vi "Write StreamChannels.vi"(8 "error in (no error)":errorcluster, 10 "StreamChannels":string[](array[string]), 11 "WaveformAcq configuration in":refnum<class "WaveformAcq configuration.lvclass">) -> (0 "error out":errorcluster, 3 "WaveformAcq configuration out":refnum<class "WaveformAcq configuration.lvclass">)   [LabVIEW 2017, in "WaveformAcq configuration.lvclass"]
uses:
  WaveformAcq configuration.lvclass
  WaveformAcq configuration.lvclass/WaveformAcq configuration.ctl
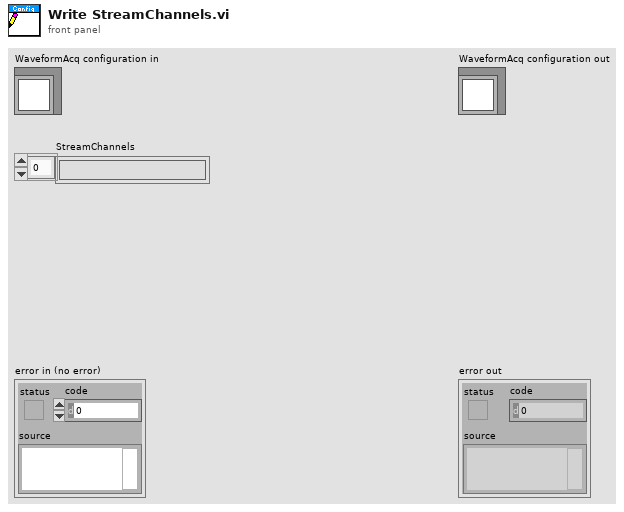
[diagram p1: front panel]
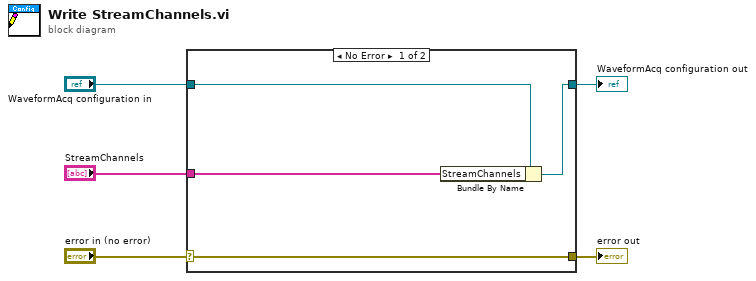
[diagram p0: block diagram]
diagram:
  n1 = case shown="No Error" "error in (no error)" {
    selector: "error in (no error)" -> [w9 w10]
    tunnel: [w9 w10] -> w4
    tunnel: [w7 w11] -> w2
    tunnel: "WaveformAcq configuration in" -> [w8 w11]
    tunnel: "StreamChannels" -> [w6 _]
    frame No Error {
      n2 = Bundle By Name(cluster=w8, "StreamChannels"=w6) -> (w7:refnum<class "WaveformAcq configuration.lvclass">)
    }
    frame Error {
    }
  }
  "error out" <- w4
  "WaveformAcq configuration out" <- w2
